vi "LVClass_WavefrontCorrectorSet Get Parameter Type.vi"(0 "WavefrontCorrectorSet in":refnum<class "WavefrontCorrectorSet.lvclass">, 5 "parameter_name":string, 11 "error in (no error)":errorcluster) -> (4 "WavefrontCorrectorSet out":refnum<class "WavefrontCorrectorSet.lvclass">, 6 "Type":T1, 15 "error out":errorcluster)   [LabVIEW 2020, in "WavefrontCorrectorSet.lvclass"]
doc: "WavefrontCorrector parameter type getter given its name which should have been\nread with Imop_WavefrontCorrectorSet_GetParameterName.\n\n--------------------------------------------------------------------------------\n\n<B>wavefrontcorrector_setIn </B> : WavefrontCorrectorSet object.\n<B>wavefrontcorrector_setOut </B> : WavefrontCorrectorSet object.\n<B>parameter_name </B> : Parameter name.\n<B>type </B> : Parameter type.\n<B>ErrorIn </B> : Error\n<B>ErrorOut </B> : Error\n\n--------------------------------------------------------------------------------"
uses:
  WavefrontCorrectorSet.lvclass
  CameraParameters_Type.ctl
  WavefrontCorrectorSet.lvclass/WavefrontCorrectorSet.ctl
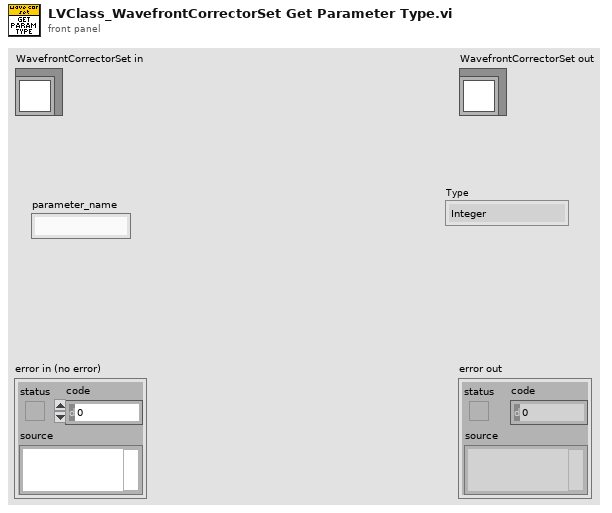
[diagram p1: front panel]
types:
  T1 = typedef "CameraParameters_Type.ctl" = enum16{"Integer", "Real", "String", "Boolean"}
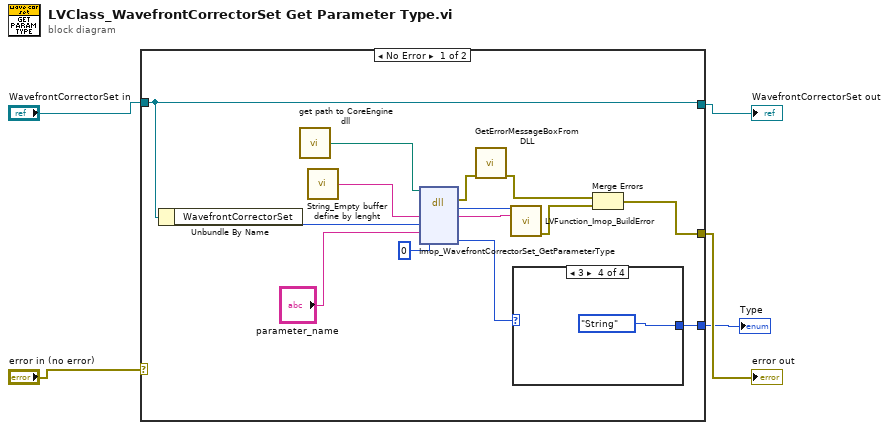
[diagram p0: block diagram]
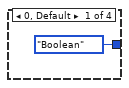
[diagram p2: hidden frame]
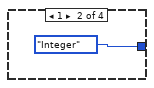
[diagram p3: hidden frame]
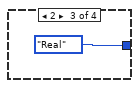
[diagram p4: hidden frame]
diagram:
  n1 = case shown="No Error" "error in (no error)" {
    selector: "error in (no error)" -> [_ w24]
    tunnel: "WavefrontCorrectorSet in" -> [w6 w25]
    tunnel: [w6 w25] -> w3
    tunnel: [w7 w24] -> w2
    tunnel: [w11 _] -> w1
    frame No Error {
      n2 = Unbundle By Name(w6) -> ("WavefrontCorrectorSet"=w10:i32)
      n3 = call "get path to CoreEngine dll.vi"() -> ("path to c_interface_vc100.dll"=w14:path)  [unwired: 12 in, 3 out]
      n4 = call "String_Empty buffer define by lenght.vi"() -> ("Empty buffer"=w17:string)  [unwired: 1 in]
      n5 = dll-call lib="D:/soft/HASO_v3/C_interface/Sources/Build/vc100/Release/c_interface_vc100.dll" fn="Imop_WavefrontCorrectorSet_GetParameterType"(path in=w14, "message"=w17, "objet"=w10, "parameter_name"="parameter_name", "type"=u32 0) -> (error out=w13:errorcluster, "return type"=w19:i32, "message"=w18:string, "type"=w12:i32)  [unwired: 4 in, 1 out]
      n6 = call "GetErrorMessageBoxFromDLL.vi"("error IN"=w13) -> ("error OUT"=w9:errorcluster)  [unwired: 10 in]
      n7 = call "LVFunction_Imop_BuildError.vi"("code"=w19, "String to Prepend to source (\"\")"=w18) -> ("error out"=w8:errorcluster)  [unwired: 13 in]
      n8 = case shown="3" w12 {
        tunnel: [CameraParameters_Type."Boolean" ("Type 2") CameraParameters_Type."Integer" ("Type 2") CameraParameters_Type."Real" ("Type 2") CameraParameters_Type."String" ("Type 2")] -> w11
        frame 0, Default {
        }
        frame 1 {
        }
        frame 2 {
        }
        frame 3 {
        }
      }
      n9 = Merge Errors(w9, w8) -> (w7:errorcluster)
    }
    frame Error {
    }
  }
  "error out" <- w2
  "WavefrontCorrectorSet out" <- w3
  "Type" <- w1
